vi "Convert Counter Value TIO 2.vi"(8 "Rollovers":u32, 10 "Last Time of Arrival (counts)":u32, 11 "Time of Arrival (counts)":u32) -> (0 "Rollovers Out":u32, 3 "Reverse Order":bool)   [LabVIEW 2009]
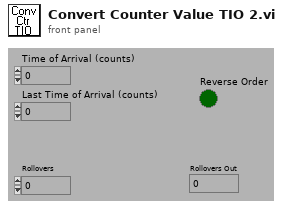
[diagram p1: front panel]
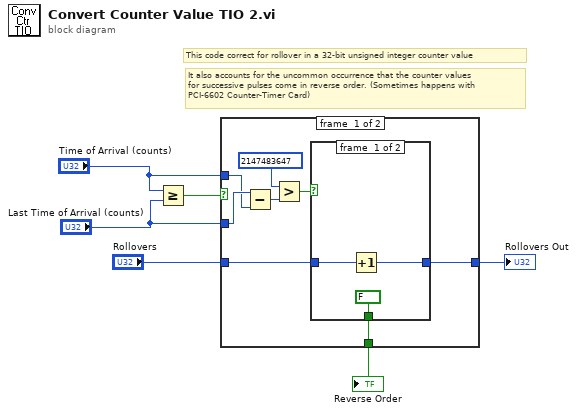
[diagram p0: block diagram]
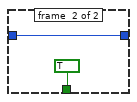
[diagram p2: hidden frame]
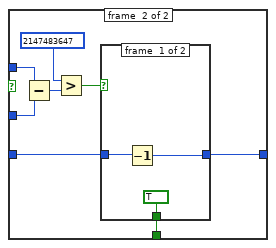
[diagram p3: hidden frame]
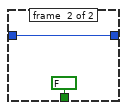
[diagram p4: hidden frame]
diagram:
  # "It also accounts for the uncommon occurrence that the counter values\nfor successive pulses come in reverse order. (Sometimes happens with\nPCI-6602 Counter-Timer Card)"
  # "This code correct for rollover in a 32-bit unsigned integer counter value"
  n1 = Greater Or Equal?(x="Time of Arrival (counts)", y="Last Time of Arrival (counts)") -> (x >= y?=w6:bool)
  n2 = case shown="False" w6 {
    tunnel: "Time of Arrival (counts)" -> [w8 w22]
    tunnel: "Last Time of Arrival (counts)" -> [w9 w21]
    tunnel: "Rollovers" -> [w12 w24]
    tunnel: [w11 w23] -> w3
    tunnel: [w7 w20] -> w1
    frame #0 {
      n3 = Subtract(x=w9, y=w8) -> (x-y=w10:u32)
      n4 = Greater?(x=u32 2147483647, y=w10) -> (0:w13:bool)
      n5 = case shown="True" w13 {
        tunnel: w12 -> [w17 w19]
        tunnel: [w16 w19] -> w11
        tunnel: [FALSE TRUE] -> w7
        frame #0 {
          n6 = Increment(x=w17) -> (x+1=w16:u32)
        }
        frame #1 {
        }
      }
    }
    frame #1 {
      n7 = Subtract(x=w22, y=w21) -> (x-y=w26:u32)
      n8 = Greater?(x=u32 2147483647, y=w26) -> (0:w25:bool)
      n9 = case shown="False" w25 {
        tunnel: w24 -> [w30 w32]
        tunnel: [w29 w32] -> w23
        tunnel: [TRUE FALSE] -> w20
        frame #0 {
          n10 = Decrement(x=w30) -> (x-1=w29:u32)
        }
        frame #1 {
        }
      }
    }
  }
  "Rollovers Out" <- w3
  "Reverse Order" <- w1
